vi "PID_subvi.vi"() -> ()   [LabVIEW 2013]
uses:
  <vilib>/myRIO/Instrument Drivers/Onboard IO/AO/vis/Smart Open.vi
  <vilib>/myRIO/Instrument Drivers/Onboard IO/AO/vis/Write.vi
  <vilib>/myRIO/Instrument Drivers/Onboard IO/AO/vis/Open.vi
  <vilib>/myRIO/Common/Instrument Driver Framework/myRIO v1.0/AO/vis/myRIO v1.1 Open AO.vi
  <vilib>/myRIO/Common/Instrument Driver Framework/Utilities/vis/Validate Channels.vi
  <vilib>/myRIO/Common/Instrument Driver Framework/myRIO v1.0/AO/vis/myRIO v1.0 Reserve AO.vi
  <vilib>/myRIO/Common/Instrument Driver Framework/myRIO v1.0/AO/vis/myRIO v1.0 Build MUX Configuration AO.vi
  <vilib>/myRIO/Common/Instrument Driver Framework/myRIO v1.0/Resource Manager/vis/myRIO v1.0 Reserve Channel List.vi
  <vilib>/myRIO/Common/Instrument Driver Framework/myRIO v1.0/Resource Manager/vis/myRIO v1.0 Reserve Channel.vi
  <vilib>/myRIO/Common/Instrument Driver Framework/myRIO v1.0/Resource Manager/vis/myRIO v1.0 Unreserve Channel.vi
  <vilib>/myRIO/Common/Instrument Driver Framework/myRIO v1.0/Resource Manager/vis/myRIO v1.0 Build Mutex Name.vi
  <vilib>/myRIO/Common/Instrument Driver Framework/myRIO v1.0/myRIO v1.1 Open.vi
  <vilib>/myRIO/Common/Instrument Driver Framework/myRIO v1.0/AO/vis/myRIO v1.0 Get Scaling Constants AO.vi
  <vilib>/Utility/VariantDataType/GetNumericInfo.vi
  <vilib>/Utility/error.llb/Error Cluster From Error Code.vi
  <vilib>/myRIO/Common/Instrument Driver Framework/Utilities/vis/IO Manager.vi
  <vilib>/myRIO/Common/Instrument Driver Framework/Utilities/vis/Configuration Manager.vi
  <vilib>/myRIO/Common/Instrument Driver Framework/myRIO v1.0/myRIO v1.0 Close.vi
  <vilib>/myRIO/Common/Instrument Driver Framework/myRIO v1.0/AO/vis/myRIO v1.0 Write AO.vi
panel:
  in  "KD":dbl
  in  "Initial feedback":dbl
  in  "KI":dbl=1.2
  in  "KP":dbl=1.2
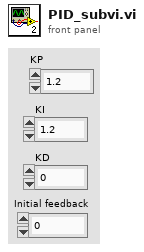
[diagram p1: front panel]
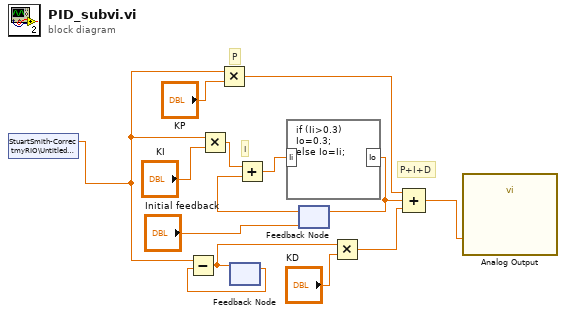
[diagram p0: block diagram]
diagram:
  # "P+I+D"
  # "P"
  # "I"
  n1 = shared-variable "StuartSmith-CorrectmyRIO\\Untitled Library 2.lvlib\\Error"() -> (w2:dbl)  [unwired: 1 in, 1 out]
  n2 = Multiply(x=w2, y="KI") -> (x*y=w13:dbl)
  n3 = Multiply(x=w2, y="KP") -> (x*y=w9:dbl)
  n4 = feedback #1() -> (w4:dbl)  [unwired: 1 in]
  n5 = Subtract(x=w2, y=w4) -> (x-y=w6:dbl)
  n6 = feedback-in #1(w6) -> ()
  n7 = feedback #2("Initial feedback") -> (w12:dbl)
  n8 = Add(x=w13, y=w12) -> (x+y=w10:dbl)
  n9 = formula code="if (Ii>0.3)\nIo=0.3;\nelse Io=Ii;"("Ii"=w10) -> ("Io"=w8:dbl)
  n10 = feedback-in #2(w8) -> ()
  n11 = Multiply(x=w6, y="KD") -> (x*y=w7:dbl)
  n12 = Compound Arithmetic op=ADD(w9, w8, w7) -> (w1:dbl)
  n13 = call "Analog Output"("A/AO0 (Pin 2)"=w1) -> ()  [unwired: 26 in, 1 out]
